vi "Simulated Temperature.vi"(1 "Lower Limit (20)":dbl=20.0, 2 "Upper Limit (30)":dbl=30.0) -> (0 "Temperature Value":dbl format="%.1g")   [LabVIEW 2017]
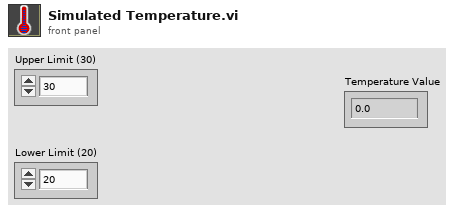
[diagram p1: front panel]
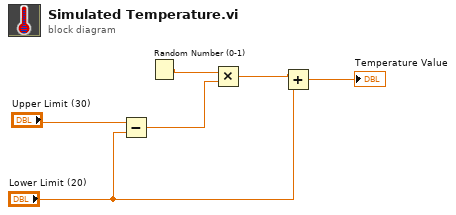
[diagram p0: block diagram]
diagram:
  n1 = Subtract(x="Upper Limit (30)", y="Lower Limit (20)") -> (x-y=w3:dbl)
  n2 = Random Number (0-1)() -> (number: 0 to 1=w6:dbl)
  n3 = Multiply(x=w6, y=w3) -> (x*y=w5:dbl)
  n4 = Add(x=w5, y="Lower Limit (20)") -> (x+y=→"Temperature Value":dbl)
